vi "PtByPt and Array Based Filter - DFD.vi"() -> ()   [LabVIEW 2023]
doc: "Compares point-by-point filtering with array-based filtering. The point-by-point filtering works in real-time and online, while the array-based filtering waits for the array to be compiled first. The example uses processing VIs in the LabVIEW Digital Filter Design Toolkit."
uses:
  <vilib>/addons/Digital Filter Design/Process.llb/DFD Filtering (PtByPt).vi
  <vilib>/addons/Digital Filter Design/Process.llb/DFD Filtering (Array).vi
  <vilib>/ptbypt/NI_PtbyPt.lvlib
  <vilib>/addons/Digital Filter Design/NI_DigFilterLicensed.lvlib
panel:
  in  "Initialize":bool=TRUE
  out "Signal (sine plus noise)":dbl(graph)=1.0271080859911303
  out "Filtered Signal \nArray Based":dbl[](graph) caption="Filtered Signal Array Based"
  in  "Stop":bool
  out "Filtered Signal Point-By-Point":dbl(graph)=1.0726722873935919
  # "Select Help»Show Context Help and move the cursor over the VI icon for more information."
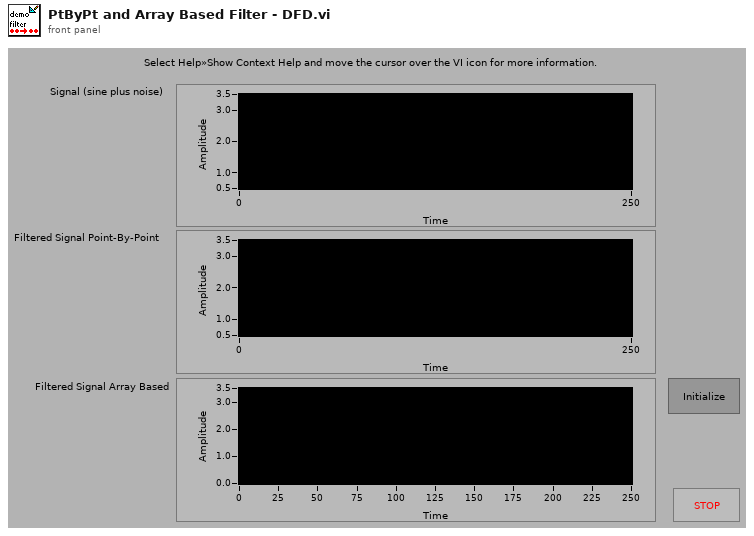
[diagram p1: front panel]
types:
  T1 = typedef "NI_DigFilterLicensed.lvlib/DFD Filter Obj.ctl" = cluster{"mSRate_Fs":dbl, "mSRate_Version":string, "mSRate_Comments":string, "mSRate_OrgCoef":T2, "mSRate_CurCoef":T2, "mSRate_Quantized?":bool, "mSRate_QCoef":T2, "mSRate_QSettings":T4[], "mSRate_Order":i32, "mSRate_Scaling":cluster{"mSRate_ScaleByPowerOf2?":bool, "mSRate_ScaleType":T6}}
  T2 = typedef "NI_DigFilterLicensed.lvlib/DFD Filter Coef.ctl" = cluster{"type":T3, "gain":dbl, "coef a (k)":dbl[], "coef b (v)":dbl[]}
  T3 = typedef "NI_DigFilterLicensed.lvlib/DFD Filter Structure Type Selector.ctl" = enum16{"Undefined", "FIR Direct Form", "FIR Direct Form Transposed", "FIR Symmetric", "FIR Antisymmetric", "IIR Direct Form I", "IIR Direct Form I Transposed", "IIR Direct Form II", "IIR Direct Form II Transposed", "IIR Cascaded Second Order Sections Form I", "IIR Cascaded Second Order Sections Form I Transposed", "IIR Cascaded Second Order Sections Form II", "IIR Cascaded Second Order Sections Form II Transposed", "Lattice Allpass (basic sections)", "Lattice Allpass (one multiplier sections)", "Lattice Allpass (normalized sections)", "Lattice AR (basic sections)", "Lattice AR (one multiplier sections)", "Lattice AR (normalized sections)", "Lattice MA (minimum phase)", "Lattice MA (maximum phase)", "Lattice ARMA (basic sections)", "Lattice ARMA (one multiplier sections)", "Lattice ARMA (normalized sections)"}
  T4 = typedef "NI_DigFilterLicensed.lvlib/dfd_Internal Quantization Settings.ctl" = cluster{"source":T5, "wl":i16, "iwl":i16, "overflow mode":enum16{"Saturation", "Wrap"}, "rounding mode":enum16{"Nearest", "Truncation"}, "signed?":bool}
  T5 = typedef "NI_DigFilterLicensed.lvlib/dfd_Internal Quantization Srcs.ctl" = u16
  T6 = typedef "NI_DigFilterLicensed.lvlib/DFD Coef Norm Type.ctl" = enum16{"No Norm", "Time Domain 1-Norm", "Time Domain 2-Norm", "Time Domain Inf-Norm"}
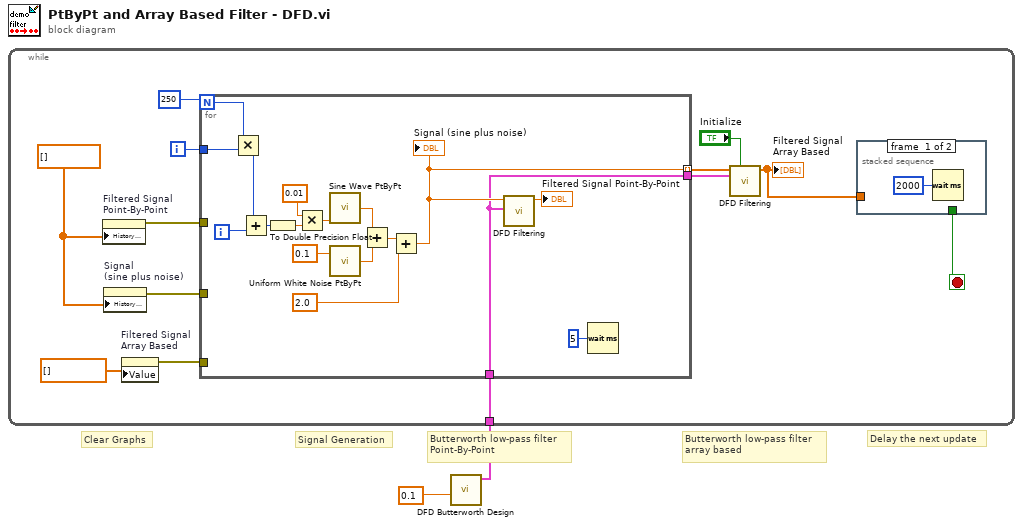
[diagram p0: block diagram]
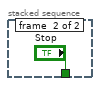
[diagram p2: hidden frame]
diagram:
  # "Delay the next update"
  # "Clear Graphs"
  # "Butterworth low-pass filter\narray based"
  # "Butterworth low-pass filter\nPoint-By-Point"
  # "Signal Generation"
  n1 = call <vilib>:"DFD Butterworth Design.vi"("low cutoff freq [Hz]"=0.1 ("low cutoff freq: fl")) -> ("filter out"=w1:T1)  [unwired: 5 in, 5 out]
  n2 = while {
    tunnel: w1 -> [w3]
    i -> [w14]
    stop <- w13 stop-if-true
    w11 = dbl[] [] ("Output Array")
    n3 = property on="Filtered Signal \nPoint-By-Point" class="WFChart (strict)"("History Data"=w11) -> (error out=w10:errorcluster)  [unwired: 2 in, 1 out]
    n4 = property on="Signal \n(sine plus noise)" class="WFChart (strict)"("History Data"=w11) -> (error out=w9:errorcluster)  [unwired: 2 in, 1 out]
    n5 = property on="Filtered Signal \nArray Based" class="WFGraph (strict)"("Value"=dbl[] [] ("Filtered Signal Array Based")) -> (error out=w8:errorcluster)  [unwired: 2 in, 1 out]
    n6 = for {
      N: 250 -> [w26]
      tunnel: [w20] -> w7 mode=indexing
      tunnel: w14 -> [w25]
      tunnel: w10 -> [_]
      tunnel: w9 -> [_]
      tunnel: w8 -> [_]
      tunnel: [w18] -> w5
      tunnel: w3 -> [w18]
      i -> [w34]
      n7 = Multiply(x=w26, y=w25) -> (x*y=w24:i32)
      n8 = Add(x=w24, y=w34) -> (x+y=w22:i32)
      n9 = To Double Precision Float(number=w22) -> (double precision float=w21:dbl)
      n10 = Multiply(x=0.01, y=w21) -> (x*y=w31:dbl)
      n11 = call <vilib>:"Sine Wave PtByPt.vi"("time"=w31) -> ("sine wave"=w33:dbl)  [unwired: 3 in]
      n12 = call <vilib>:"Uniform White Noise PtByPt.vi"("amplitude"=0.1) -> ("uniform white noise"=w32:dbl)  [unwired: 2 in]
      n13 = Add(x=w33, y=w32) -> (x+y=w27:dbl)
      n14 = Add(x=w27, y=2.0) -> (x+y=w20:dbl)
      "Signal (sine plus noise)" <- w20
      n15 = call-poly <vilib>:"DFD Filtering.vi"("filter"=w18, "signal in"=w20) -> ("signal out"=→"Filtered Signal Point-By-Point":dbl)  [unwired: 2 in, 7 out]
      n16 = Wait (ms)(milliseconds to wait=u32 5) -> ()  [unwired: 1 out]
    }
    n17 = call-poly <vilib>:"DFD Filtering.vi"("init? (F)"="Initialize", "filter"=w5, "signal in"=w7) -> ("signal out"=w6:dbl[])  [unwired: 1 in, 7 out]
    "Filtered Signal \nArray Based" <- w6
    n18 = stacked-sequence {
      tunnel: w6 -> [_ _]
      tunnel: [_ "Stop"] -> w13
      frame #0 {
        n19 = Wait (ms)(milliseconds to wait=u32 2000) -> ()  [unwired: 1 out]
      }
      frame #1 {
      }
    }
  }
